vi "GetClimbSpeed.vi"(11 "Climber in":refnum<class "Climber.lvclass">) -> (2 "Climb Speed":dbl, 3 "Climber out":refnum<class "Climber.lvclass">)   [LabVIEW 2016, in "Climber.lvclass"]
uses:
  Climber.lvclass
  Climber.lvclass/Climber.ctl
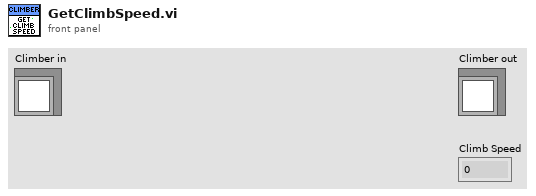
[diagram p1: front panel]
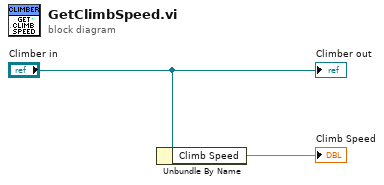
[diagram p0: block diagram]
diagram:
  n1 = Unbundle By Name("Climber in") -> ("Climb Speed"=→"Climb Speed":dbl)
  "Climber out" <- "Climber in"
